vi "dfd_FXP PtByPt Lattice ARMA (normalized).vi"(0 "x":T7={"value"=0, "wl"=0, "iwl"=0, "Signed"=TRUE} {"value" format="%.0x"}, 1 "coef k[M..1]":T1, 2 "coef ^k[M..1]":T1, 3 "coef v[M..0]":T1, 5 "filtering statistics in":T4(array[cluster]) {"statistics information"."min value" format="%.2f"; "statistics information"."max value" format="%.2f"; "Quantizer Source" items=["Coefficients a/k"=0, "Coefficients b/v"=7, "Input"=1, "Output"=2, "Multiplicand"=3, "Product"=4, "Sum"=5, "Delay"=6]}, 6 "FXPOPs":T5[](array[typedef]) {"source" items=["Coef a/k"=0, "Coef b/v"=7, "Input"=1, "Output"=2, "Multiplicand"=3, "Product"=4, "Sum"=5, "Delay"=6, "Gain"=8]}, 9 "state in":i64[](array[numeric])) -> (11 "state out":i64[](array[numeric]), 14 "filtered x":T7={"value"=0, "wl"=0, "iwl"=0, "Signed"=TRUE} {"value" format="%.0x"}, 19 "filtering statistics out":T4(array[cluster]) {"statistics information"."min value" format="%.2f"; "statistics information"."max value" format="%.2f"; "Quantizer Source" items=["Coefficients a/k"=0, "Coefficients b/v"=7, "Input"=1, "Output"=2, "Multiplicand"=3, "Product"=4, "Sum"=5, "Delay"=6]})   [LabVIEW 2017, in "NI_DigFilter_FXP.lvlib"]
uses:
  <vilib>/addons/Digital Filter Design/NI_DigFilter_FXP.lvlib
  <vilib>/addons/Digital Filter Design/_Objects.llb/dfd_DFXP Data Type (scaler).ctl
  <vilib>/addons/Digital Filter Design/_Objects.llb/dfd_DFXP Operation Parameter.ctl
  <vilib>/addons/Digital Filter Design/_Objects.llb/dfd_Internal Quantization Srcs.ctl
  <vilib>/addons/Digital Filter Design/_Objects.llb/dfd_DFXP Data Type (vector).ctl
  <vilib>/addons/Digital Filter Design/_Objects.llb/DFD Quantization Sources.ctl
  <vilib>/addons/Digital Filter Design/_Objects.llb/DFD FXP Statistics Data.ctl
  <vilib>/addons/Digital Filter Design/NI_DigFilterLicensed.lvlib
panel:
  in  "DFXP array type":T1
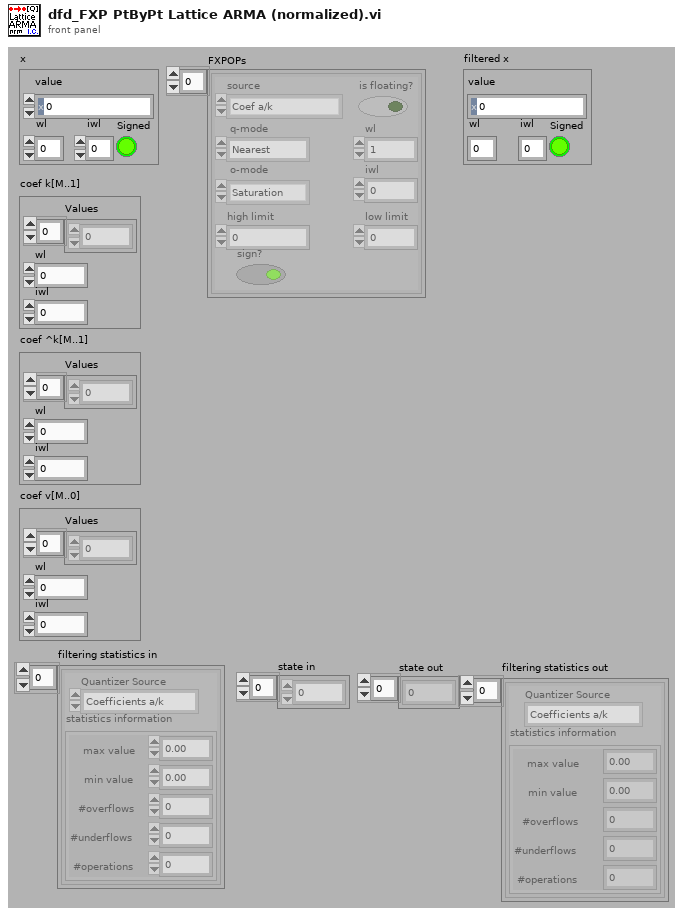
[diagram p1: front panel]
types:
  T1 = typedef "dfd_DFXP Data Type (vector).ctl" = cluster{"Values":i64[], "wl":i16, "iwl":i16}
  T2 = typedef "NI_DigFilterLicensed.lvlib/DFD Quantization Sources.ctl" = u16
  T3 = typedef "NI_DigFilterLicensed.lvlib/DFD FXP Statistics Data.ctl" = cluster{"max value":ext, "min value":ext, "#overflows":i32, "#underflows":i32, "#operations":i32}
  T4 = cluster{"Quantizer Source":T2, "statistics information":T3}[]
  T5 = typedef "dfd_DFXP Operation Parameter.ctl" = cluster{"source":T6, "is floating?":bool, "o-mode":enum16{"Saturation", "Wrap"}, "q-mode":enum16{"Nearest", "Truncation"}, "wl":i16, "high limit":i64, "low limit":i64, "iwl":i16, "sign?":bool}
  T6 = typedef "NI_DigFilterLicensed.lvlib/dfd_Internal Quantization Srcs.ctl" = u16
  T7 = typedef "dfd_DFXP Data Type (scaler).ctl" = cluster{"value":i64, "wl":i16, "iwl":i16, "Signed":bool}
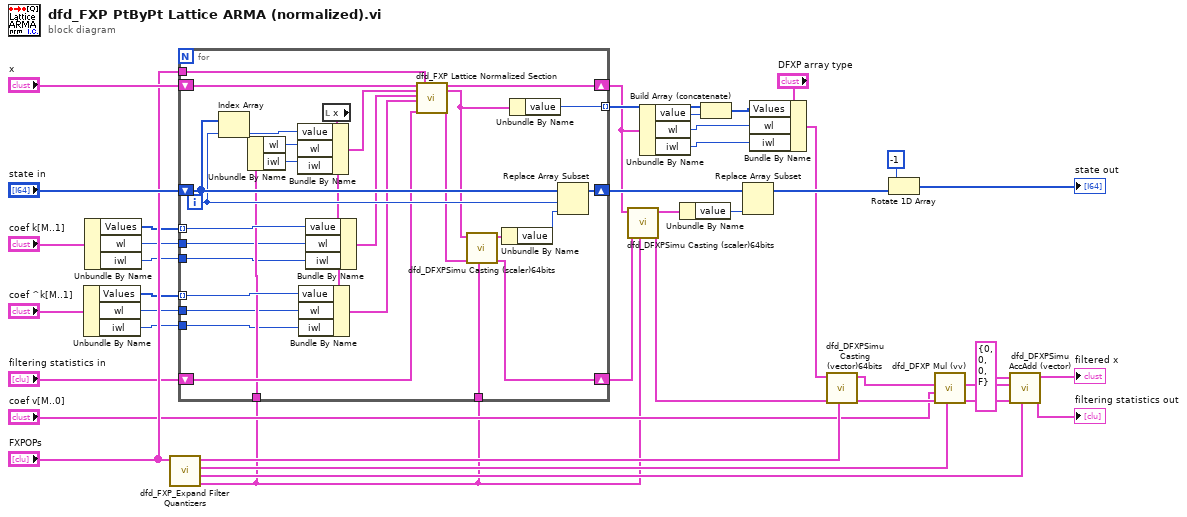
[diagram p0: block diagram]
diagram:
  n1 = Unbundle By Name("coef ^k[M..1]") -> ("Values"=w9:i64[], "wl"=w8:i16, "iwl"=w7:i16)
  n2 = Unbundle By Name("coef k[M..1]") -> ("Values"=w12:i64[], "wl"=w11:i16, "iwl"=w10:i16)
  n3 = call <vilib>:"dfd_FXP_Expand Filter Quantizers.vi"("FXPOPs"="FXPOPs") -> ("Delay"=w13:T5, "Sum"=w19:T5, "Product"=w22:T5, "Multiplicand"=w24:T5)  [unwired: 7 out]
  n4 = for {
    shift-right: [w60] -> w28
    shift-left: "x" -> [w64]
    tunnel: w9 -> [w61] mode=indexing
    shift-right: [w67] -> w35
    shift-left: "state in" -> [w68]
    tunnel: w12 -> [w62] mode=indexing
    tunnel: w13 -> [w56]
    tunnel: "FXPOPs" -> [w59]
    shift-right: [w58] -> w27
    shift-left: "filtering statistics in" -> [w54]
    tunnel: [w41] -> w29 mode=indexing
    tunnel: w13 -> [w52]
    tunnel: w11 -> [w48]
    tunnel: w10 -> [w47]
    tunnel: w8 -> [w44]
    tunnel: w7 -> [w43]
    i -> [w66]
    n5 = Index Array(array=w68, index=w66) -> (element=w63:i64)
    n6 = Unbundle By Name(w52) -> ("wl"=w51:i16, "iwl"=w50:i16)
    n7 = local read "x"() -> (w45:T7)
    n8 = Bundle By Name(cluster=w45, "value"=w63, "wl"=w51, "iwl"=w50) -> (w53:T7)
    n9 = Bundle By Name(cluster=w45, "value"=w61, "wl"=w44, "iwl"=w43) -> (w46:T7)
    n10 = Bundle By Name(cluster=w45, "value"=w62, "wl"=w48, "iwl"=w47) -> (w49:T7)
    n11 = call <vilib>:"dfd_FXP Lattice Normalized Section.vi"("x(m)"=w64, "w(m-1)"=w53, "k(m)"=w49, "^k(m)"=w46, "filtering statistics in"=w54, "FXPOPs"=w59) -> ("x(m-1)"=w60:T7, "w(m)"=w55:T7, "filtering statistics out"=w57:T4)  [unwired: 11 out]
    n12 = call <vilib>:"dfd_DFXPSimu Casting (scaler)64bits.vi"("op params"=w56, "filtering statistics in"=w57, "Value in"=w55) -> ("filtering statistics out"=w58:T4, "Value out"=w65:T7)  [unwired: 2 in, 5 out]
    n13 = Unbundle By Name(w65) -> ("value"=w42:i64)
    n14 = Unbundle By Name(w55) -> ("value"=w41:i64)
    n15 = Replace Array Subset(array=w68, new element=w42, index=w66) -> (w67:i64[])
  }
  n16 = call <vilib>:"dfd_DFXPSimu Casting (scaler)64bits.vi"("op params"=w13, "filtering statistics in"=w27, "Value in"=w28) -> ("filtering statistics out"=w25:T4, "Value out"=w34:T7)  [unwired: 2 in, 5 out]
  n17 = Unbundle By Name(w28) -> ("value"=w6:i64, "wl"=w2:i16, "iwl"=w1:i16)
  n18 = Unbundle By Name(w34) -> ("value"=w5:i64)
  n19 = Build Array (concatenate)(w29, w6) -> (w26:i64[])
  n20 = Replace Array Subset(array=w35, new element=w5) -> (w33:i64[])  [unwired: 1 in]
  n21 = Bundle By Name(cluster="DFXP array type", "Values"=w26, "wl"=w2, "iwl"=w1) -> (w4:T1)
  n22 = call <vilib>:"dfd_DFXPSimu Casting (vector)64bits.vi"("op params"=w24, "filtering statistics in"=w25, "Value in"=w4) -> ("filtering statistics out"=w23:T4, "Value out"=w16:T1)  [unwired: 1 in, 6 out]
  n23 = Rotate 1D Array(1:w33, 2:-1 ("n")) -> (0:→"state out":i64[])
  n24 = call <vilib>:"dfd_DFXP Mul (vv).vi"("op params"=w22, "filtering statistics in"=w23, "Value in 2"="coef v[M..0]", "Value in"=w16) -> ("filtering statistics out"=w21:T4, "Value out"=w20:T1)  [unwired: 6 out]
  n25 = call <vilib>:"dfd_DFXPSimu AccAdd (vector).vi"("op params"=w19, "filtering statistics in"=w21, "addends"=w20, "acc in"=T7 {"value"=0, "wl"=0, "iwl"=0, "Signed"=FALSE}) -> ("filtering statistics out"=→"filtering statistics out":T4, "acc out"=→"filtered x":T7)  [unwired: 1 in, 5 out]
